vi "ASIC_Selecor canal Sumador (func sumas).vi"(7 "Espera acceso USB":u32=10, 8 "error in":errorcluster, 9 "Sumador":u8, 10 "Modo":u8, 11 "ftHandle_in":u32) -> (0 "error out":errorcluster, 1 "N sumadores":u8, 2 "Reg 101-100":u32, 3 "ftHandle_out":u32)   [LabVIEW 2019]
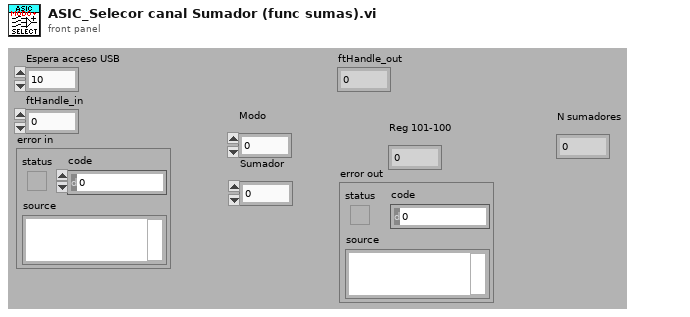
[diagram p1: front panel]
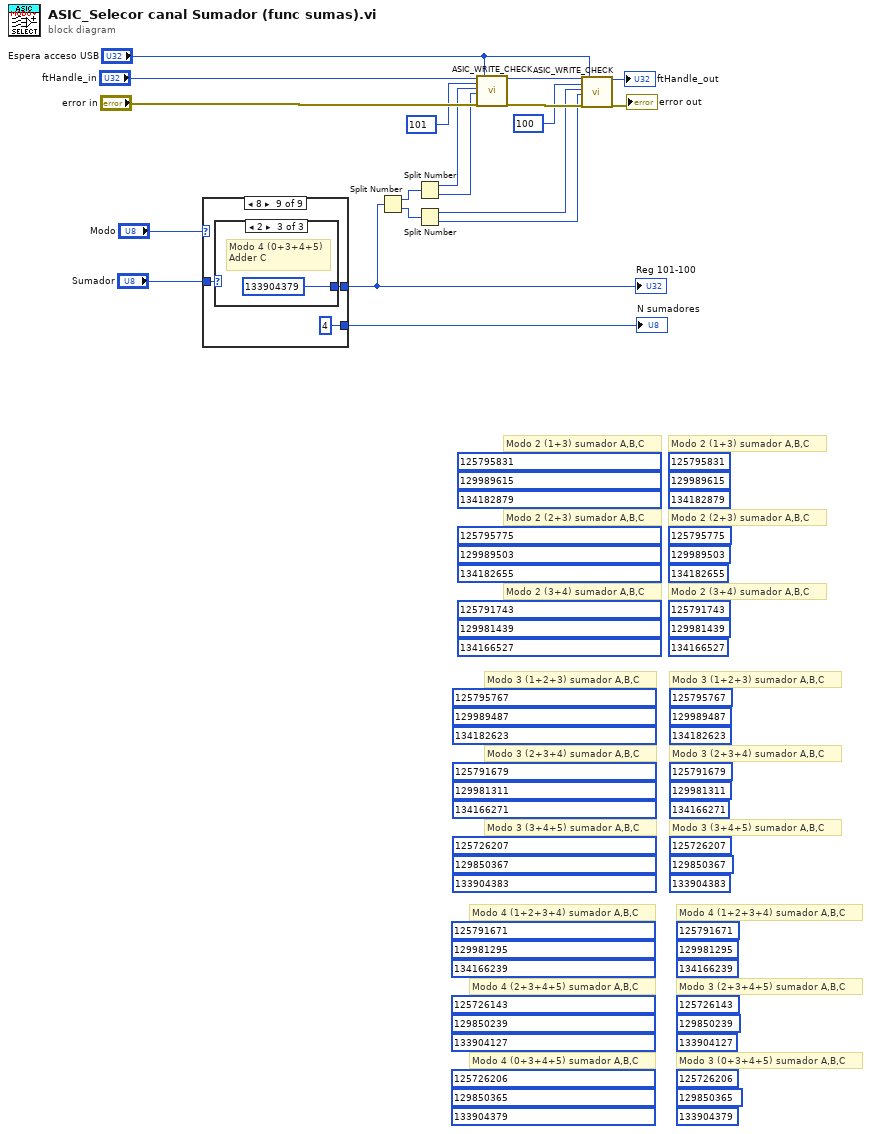
[diagram p0: block diagram]
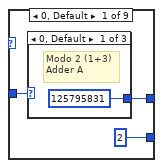
[diagram p2: hidden frame]
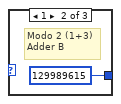
[diagram p3: hidden frame]
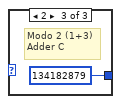
[diagram p4: hidden frame]
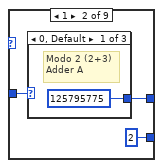
[diagram p5: hidden frame]
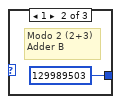
[diagram p6: hidden frame]
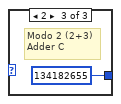
[diagram p7: hidden frame]
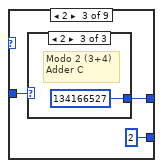
[diagram p8: hidden frame]
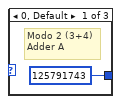
[diagram p9: hidden frame]
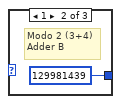
[diagram p10: hidden frame]
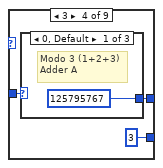
[diagram p11: hidden frame]
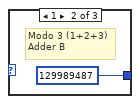
[diagram p12: hidden frame]
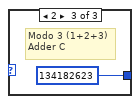
[diagram p13: hidden frame]
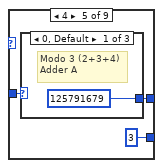
[diagram p14: hidden frame]
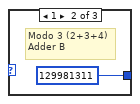
[diagram p15: hidden frame]
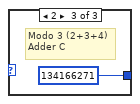
[diagram p16: hidden frame]
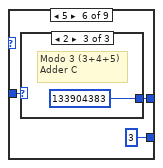
[diagram p17: hidden frame]
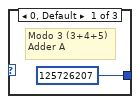
[diagram p18: hidden frame]
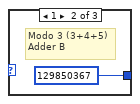
[diagram p19: hidden frame]
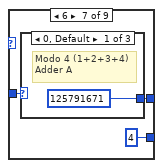
[diagram p20: hidden frame]
diagram:
  (unwired) u32 133904379 ("Threshold Inicial N")
  (unwired) u32 129850365 ("Threshold Inicial N")
  (unwired) u32 125726206 ("Threshold Inicial N")
  (unwired) u32 133904127 ("Threshold Inicial N")
  (unwired) u32 129850239 ("Threshold Inicial N")
  (unwired) u32 125726143 ("Threshold Inicial N")
  (unwired) u32 134166239 ("Threshold Inicial N")
  (unwired) u32 129981295 ("Threshold Inicial N")
  (unwired) u32 125791671 ("Threshold Inicial N")
  (unwired) u32 133904379 ("Threshold Inicial N")
  (unwired) u32 129850365 ("Threshold Inicial N")
  (unwired) u32 125726206 ("Threshold Inicial N")
  (unwired) u32 133904127 ("Threshold Inicial N")
  (unwired) u32 129850239 ("Threshold Inicial N")
  (unwired) u32 125726143 ("Threshold Inicial N")
  (unwired) u32 134166239 ("Threshold Inicial N")
  (unwired) u32 129981295 ("Threshold Inicial N")
  (unwired) u32 125791671 ("Threshold Inicial N")
  (unwired) u32 133904383 ("Threshold Inicial N")
  (unwired) u32 129850367 ("Threshold Inicial N")
  (unwired) u32 125726207 ("Threshold Inicial N")
  (unwired) u32 134166271 ("Threshold Inicial N")
  (unwired) u32 129981311 ("Threshold Inicial N")
  (unwired) u32 125791679 ("Threshold Inicial N")
  (unwired) u32 134182623 ("Threshold Inicial N")
  (unwired) u32 129989487 ("Threshold Inicial N")
  (unwired) u32 125795767 ("Threshold Inicial N")
  (unwired) u32 133904383 ("Threshold Inicial N")
  (unwired) u32 129850367 ("Threshold Inicial N")
  (unwired) u32 125726207 ("Threshold Inicial N")
  (unwired) u32 134166271 ("Threshold Inicial N")
  (unwired) u32 129981311 ("Threshold Inicial N")
  (unwired) u32 125791679 ("Threshold Inicial N")
  (unwired) u32 134182623 ("Threshold Inicial N")
  (unwired) u32 129989487 ("Threshold Inicial N")
  (unwired) u32 125795767 ("Threshold Inicial N")
  (unwired) u32 134166527 ("Threshold Inicial N")
  (unwired) u32 129981439 ("Threshold Inicial N")
  (unwired) u32 125791743 ("Threshold Inicial N")
  (unwired) u32 134182655 ("Threshold Inicial N")
  (unwired) u32 129989503 ("Threshold Inicial N")
  (unwired) u32 125795775 ("Threshold Inicial N")
  (unwired) u32 134182879 ("Threshold Inicial N")
  (unwired) u32 129989615 ("Threshold Inicial N")
  (unwired) u32 125795831 ("Threshold Inicial N")
  (unwired) u32 134166527 ("Threshold Inicial N")
  (unwired) u32 129981439 ("Threshold Inicial N")
  (unwired) u32 125791743 ("Threshold Inicial N")
  (unwired) u32 134182655 ("Threshold Inicial N")
  (unwired) u32 129989503 ("Threshold Inicial N")
  (unwired) u32 125795775 ("Threshold Inicial N")
  (unwired) u32 134182879 ("Threshold Inicial N")
  (unwired) u32 129989615 ("Threshold Inicial N")
  (unwired) u32 125795831 ("Threshold Inicial N")
  # "Modo 3 (0+3+4+5) sumador A,B,C"
  # "Modo 3 (2+3+4+5) sumador A,B,C"
  # "Modo 4 (1+2+3+4) sumador A,B,C"
  # "Modo 4 (0+3+4+5) sumador A,B,C"
  # "Modo 4 (2+3+4+5) sumador A,B,C"
  # "Modo 4 (1+2+3+4) sumador A,B,C"
  # "Modo 3 (3+4+5) sumador A,B,C"
  # "Modo 3 (2+3+4) sumador A,B,C"
  # "Modo 3 (1+2+3) sumador A,B,C"
  # "Modo 3 (3+4+5) sumador A,B,C"
  # "Modo 3 (2+3+4) sumador A,B,C"
  # "Modo 3 (1+2+3) sumador A,B,C"
  # "Modo 2 (3+4) sumador A,B,C"
  # "Modo 2 (2+3) sumador A,B,C"
  # "Modo 2 (1+3) sumador A,B,C"
  # "Modo 2 (3+4) sumador A,B,C"
  # "Modo 2 (2+3) sumador A,B,C"
  # "Modo 2 (1+3) sumador A,B,C"
  n1 = case shown="8" "Modo" {
    tunnel: "Sumador" -> [w22 w28 w34 w40 w46 w52 w58 w64 w70]
    tunnel: [w21 w27 w33 w39 w45 w51 w57 w63 w69] -> w2
    tunnel: [u8 2 ("N sumadores") u8 2 ("N sumadores") u8 2 ("N sumadores") u8 3 ("N sumadores") u8 3 ("N sumadores") u8 3 ("N sumadores") u8 4 ("N sumadores") u8 4 ("N sumadores") u8 4 ("N sumadores")] -> w1
    frame 0, Default {
      n2 = case shown="0, Default" w22 {
        tunnel: [u32 125795831 ("Threshold Inicial N") u32 129989615 ("Threshold Inicial N") u32 134182879 ("Threshold Inicial N")] -> w21
        frame 0, Default {
          # "Modo 2 (1+3)\nAdder A"
        }
        frame 1 {
          # "Modo 2 (1+3)\nAdder B"
        }
        frame 2 {
          # "Modo 2 (1+3)\nAdder C"
        }
      }
    }
    frame 1 {
      n3 = case shown="0, Default" w28 {
        tunnel: [u32 125795775 ("Threshold Inicial N") u32 129989503 ("Threshold Inicial N") u32 134182655 ("Threshold Inicial N")] -> w27
        frame 0, Default {
          # "Modo 2 (2+3)\nAdder A"
        }
        frame 1 {
          # "Modo 2 (2+3)\nAdder B"
        }
        frame 2 {
          # "Modo 2 (2+3)\nAdder C"
        }
      }
    }
    frame 2 {
      n4 = case shown="2" w34 {
        tunnel: [u32 125791743 ("Threshold Inicial N") u32 129981439 ("Threshold Inicial N") u32 134166527 ("Threshold Inicial N")] -> w33
        frame 0, Default {
          # "Modo 2 (3+4)\nAdder A"
        }
        frame 1 {
          # "Modo 2 (3+4)\nAdder B"
        }
        frame 2 {
          # "Modo 2 (3+4)\nAdder C"
        }
      }
    }
    frame 3 {
      n5 = case shown="0, Default" w40 {
        tunnel: [u32 125795767 ("Threshold Inicial N") u32 129989487 ("Threshold Inicial N") u32 134182623 ("Threshold Inicial N")] -> w39
        frame 0, Default {
          # "Modo 3 (1+2+3)\nAdder A"
        }
        frame 1 {
          # "Modo 3 (1+2+3)\nAdder B"
        }
        frame 2 {
          # "Modo 3 (1+2+3)\nAdder C"
        }
      }
    }
    frame 4 {
      n6 = case shown="0, Default" w46 {
        tunnel: [u32 125791679 ("Threshold Inicial N") u32 129981311 ("Threshold Inicial N") u32 134166271 ("Threshold Inicial N")] -> w45
        frame 0, Default {
          # "Modo 3 (2+3+4)\nAdder A"
        }
        frame 1 {
          # "Modo 3 (2+3+4)\nAdder B"
        }
        frame 2 {
          # "Modo 3 (2+3+4)\nAdder C"
        }
      }
    }
    frame 5 {
      n7 = case shown="2" w52 {
        tunnel: [u32 125726207 ("Threshold Inicial N") u32 129850367 ("Threshold Inicial N") u32 133904383 ("Threshold Inicial N")] -> w51
        frame 0, Default {
          # "Modo 3 (3+4+5)\nAdder A"
        }
        frame 1 {
          # "Modo 3 (3+4+5)\nAdder B"
        }
        frame 2 {
          # "Modo 3 (3+4+5)\nAdder C"
        }
      }
    }
    frame 6 {
      n8 = case shown="0, Default" w58 {
        tunnel: [u32 125791671 ("Threshold Inicial N") u32 129981295 ("Threshold Inicial N") u32 134166239 ("Threshold Inicial N")] -> w57
        frame 0, Default {
          # "Modo 4 (1+2+3+4)\nAdder A"
        }
        frame 1 {
          # "Modo 4 (1+2+3+4)\nAdder B"
        }
        frame 2 {
          # "Modo 4 (1+2+3+4)\nAdder C"
        }
      }
    }
    frame 7 {
      n9 = case shown="2" w64 {
        tunnel: [u32 125726143 ("Threshold Inicial N") u32 129850239 ("Threshold Inicial N") u32 133904127 ("Threshold Inicial N")] -> w63
        frame 0, Default {
          # "Modo 4 (2+3+4+5)\nAdder A"
        }
        frame 1 {
          # "Modo 4 (2+3+4+5)\nAdder B"
        }
        frame 2 {
          # "Modo 4 (2+3+4+5)\nAdder C"
        }
      }
    }
    frame 8 {
      n10 = case shown="2" w70 {
        tunnel: [u32 125726206 ("Threshold Inicial N") u32 129850365 ("Threshold Inicial N") u32 133904379 ("Threshold Inicial N")] -> w69
        frame 0, Default {
          # "Modo 4 (0+3+4+5)\nAdder A"
        }
        frame 1 {
          # "Modo 4 (0+3+4+5)\nAdder B"
        }
        frame 2 {
          # "Modo 4 (0+3+4+5)\nAdder C"
        }
      }
    }
  }
  "Reg 101-100" <- w2
  "N sumadores" <- w1
  n11 = Split Number(x=w2) -> (hi(x)=w18:u16, lo(x)=w19:u16)
  n12 = Split Number(x=w18) -> (hi(x)=w10:u8, lo(x)=w9:u8)
  n13 = Split Number(x=w19) -> (hi(x)=w6:u8, lo(x)=w5:u8)
  n14 = call "ASIC_WRITE_CHECK.vi"("ftHandle_in"="ftHandle_in", "Direccion Registro Asic"=u8 101, "Byte Alto"=w10, "Byte Bajo"=w9, "error in"="error in", "Espera acceso USB 2"="Espera acceso USB") -> ("ftHandle_out"=w17:u32, "error out"=w16:errorcluster)  [unwired: 11 in, 1 out]
  n15 = call "ASIC_WRITE_CHECK.vi"("ftHandle_in"=w17, "Direccion Registro Asic"=u8 100, "Byte Alto"=w6, "Byte Bajo"=w5, "error in"=w16, "Espera acceso USB 2"="Espera acceso USB") -> ("ftHandle_out"=→"ftHandle_out":u32, "error out"=→"error out":errorcluster)  [unwired: 11 in, 1 out]
